vi "Gaussian-FIT.vi"() -> ()   [LabVIEW 2014]
uses:
  <vilib>/Utility/file.llb/Read From Spreadsheet File (DBL).vi
  <vilib>/Utility/file.llb/Write To Spreadsheet File (DBL).vi
  <vilib>/Analysis/NI_AALBase.lvlib
panel:
  in  "Tab Control":T1(tab)
  out "Amplitude Gaussian FIT":cluster{dbl[], dbl[]}(graph)={[6.4e-05, 5.6e-05, 4.6e-05, 6.8e-05, 7.8e-05, 7.4e-05, 9.5e-05, 0.000102, 0.000147, 0.000188, 0.000179, 0.000194, 0.000233, 0.00028, 0.000335, 0.000368, 0.000395, 0.000446, 0.000468, 0.000498, 0.000562, 0.000618, 0.000645, 0.000701, 0.000794, 0.000861, 0.000909, 0.000954, 0.001065, 0.001094, 0.001148, 0.001209, 0.0013, 0.001352, 0.001399, 0.001466, 0.001535, 0.001652, 0.001691, 0.001795, 0.001868, 0.00196, 0.00202, 0.00211, 0.00216, 0.002174, 0.002327, 0.002362, 0.002461, 0.002579, 0.002617, 0.002789, 0.002914, 0.002903, 0.003058, 0.003139, 0.003095, 0.003248, 0.003331, 0.003408, 0.003368, 0.003563, 0.003651, 0.003758, 0.003758, 0.003954, 0.003961, 0.004072, 0.004061, 0.004096, 0.004277, 0.004275, 0.004396, 0.004423, 0.004449, 0.004604, 0.004582, 0.004732, 0.004694, 0.004793, 0.004779, 0.004842, 0.004904, 0.004958, 0.004899, 0.004964, 0.005117, 0.005151, 0.005106, 0.005159, 0.005259, 0.00524, 0.005241, 0.005238, 0.005336, 0.005361, 0.005331, 0.005344, 0.005383, 0.005275, 0.00538, 0.005499, 0.005403, 0.005524, 0.00542], [82.13729352165659, 64.7849924275446, 64.78498654301572, 53.26762424681512, 53.26848684767046, 75.33492935987732, 98.57236716401128, 95.0782689280903, 106.98838926342651, 106.98830571153056, 115.68100244184599, 146.72665216048009, 163.13830277043354, 291.19836865057766, 291.1983657333123, 210.1652309953322, 210.1652442219881, 331.0652563735002, 386.4065018531679, 401.7529834685663, 430.5029627977273, 430.50296602090975, 471.5410739421762, 503.71464143125144, 517.9881482668702, 523.924898034199, 569.4214984543443, 569.4214612337393, 631.5620103806252, 655.7737694758601, 655.4855289569315, 655.4855299040236, 732.9802005633946, 766.2747596963685, 766.2747953082397, 778.1006128617066, 847.3463703094712, 878.1237605806596, 880.4301016814038, 916.1011404952861, 963.7757722908383, 990.7197405612773, 1030.0640889501683, 1030.0640536247415, 1058.8701478567225, 1058.8702047512666, 1111.6711179926594, 1111.6711847188385, 1153.6676174579575, 1235.7737499701648, 1235.773723593764, 1294.696999033421, 1332.8062134493603, 1332.8061973980577, 1409.6029130208294, 1520.9638380251768, 1502.7931626027435, 2078.3321696288353, 2130.9631611771083, 3080.5296903165968, 2867.478006984899, 3715.361825956468, 4097.6900064907, 4097.690187942468, 5707.884613662024, 8114.949905194222, 6791.547031549109, 6791.547266896523, 7366.489185680224, 10189.609439962016, 8850.977250606367, 10323.579049145412, 10393.92726685109, 13107.806221276795, 13628.609865877474, 12680.943384489134, 13203.655141195128, 16669.633175445753, 16669.633531086878, 17380.543280107122, 19592.54328706896, 17704.220065612448, 17704.21946476618, 21213.542684772063, 19802.16276737311, 24730.65246284223, 23209.70936397237, 29513.61861830476, 29513.61863160348, 22273.330376191294, 22273.32874546767, 27522.544526863705, 23565.830426930333, 26015.740961615415, 27638.42940114356, 30998.520950667462, 30998.520956690092, 34681.3207530217, 34681.32073675544, 29985.704667462593, 32493.37376081327, 34321.094245058215, 37619.55296913469, 37619.55290491994, 37256.344447207084]}
  out "Amplitude":dbl=37256.344447207084
  out "Amplitude max of Array":cluster{dbl[], dbl[]}(graph)={[6.4e-05, 5.6e-05, 4.6e-05, 6.8e-05, 7.8e-05, 7.4e-05, 9.5e-05, 0.000102, 0.000147, 0.000188, 0.000179, 0.000194, 0.000233, 0.00028, 0.000335, 0.000368, 0.000395, 0.000446, 0.000468, 0.000498, 0.000562, 0.000618, 0.000645, 0.000701, 0.000794, 0.000861, 0.000909, 0.000954, 0.001065, 0.001094, 0.001148, 0.001209, 0.0013, 0.001352, 0.001399, 0.001466, 0.001535, 0.001652, 0.001691, 0.001795, 0.001868, 0.00196, 0.00202, 0.00211, 0.00216, 0.002174, 0.002327, 0.002362, 0.002461, 0.002579, 0.002617, 0.002789, 0.002914, 0.002903, 0.003058, 0.003139, 0.003095, 0.003248, 0.003331, 0.003408, 0.003368, 0.003563, 0.003651, 0.003758, 0.003758, 0.003954, 0.003961, 0.004072, 0.004061, 0.004096, 0.004277, 0.004275, 0.004396, 0.004423, 0.004449, 0.004604, 0.004582, 0.004732, 0.004694, 0.004793, 0.004779, 0.004842, 0.004904, 0.004958, 0.004899, 0.004964, 0.005117, 0.005151, 0.005106, 0.005159, 0.005259, 0.00524, 0.005241, 0.005238, 0.005336, 0.005361, 0.005331, 0.005344, 0.005383, 0.005275, 0.00538, 0.005499, 0.005403, 0.005524, 0.00542], [161.26124644000026, 193.5661174600001, 194.12049499399996, 188.052439994, 187.1038815500002, 206.27893655000014, 214.9023718640001, 215.15528889400014, 239.98285910000016, 239.39450044600017, 243.52077844600012, 290.69092988399996, 286.0369737860001, 314.066050784, 315.1364557740003, 350.81662177400017, 350.60690978599973, 355.4613547859999, 396.0629574719999, 417.61620512000025, 449.21960901399996, 448.27930311600005, 485.6585251160001, 524.7455412300001, 534.4413229880001, 534.1995714579998, 578.1711295359999, 578.5861845659997, 653.8300735659998, 672.812892898, 667.1914465639999, 668.808947448, 760.072502448, 797.3196844379996, 798.3633899860002, 797.3925009860003, 873.8048546480001, 899.877105106, 898.7872815639998, 944.6088681139997, 981.3642943280001, 1019.0624535720001, 1060.971357664, 1060.992231784, 1088.1771207840002, 1088.534407874, 1145.5741308739998, 1145.483352786, 1187.7170187860002, 1268.7420660020002, 1268.2114752360003, 1326.707530236, 1357.539078456, 1356.7118811139999, 1559.8703811139999, 1683.961146234, 1664.65550554, 2186.310707324, 2239.269298666, 3234.030888442, 3022.4470147740003, 3763.0056222060007, 4088.9975858, 4085.75433143, 5693.3036094300005, 8105.126077335999, 6784.511360013999, 6782.972015672, 7358.951849672001, 10186.83952789, 8848.97599834, 10318.406622732, 10386.005732224, 13107.613116772, 13624.118723106, 12678.044298666, 13204.031606338, 16651.471154778003, 16650.867261876003, 17364.227872876003, 19563.959663592, 17707.432726659998, 17707.403599994, 21179.544987994, 19763.951123329996, 24694.030239784, 23186.627665368, 29478.722628468, 29479.152732235998, 22252.341288236, 22251.449526768, 27487.696026768, 23533.155386450002, 25981.78765043, 27605.285719208, 30964.39573809, 30963.588929446, 34651.51037444601, 34650.704051236, 29954.514495236, 32468.594379241997, 34291.851381780005, 37593.372641236, 37593.324096766, 37229.240762766]}
  in  "Laser Rate (Hz)":dbl=20.0
  out "Amplitude Gaussian FIT 2":cluster{dbl[], dbl[]}(graph)={[3.2e-06, 2.8e-06, 2.3e-06, 3.4e-06, 3.9e-06, 3.6999999999999997e-06, 4.75e-06, 5.1e-06, 7.35e-06, 9.4e-06, 8.949999999999999e-06, 9.7e-06, 1.165e-05, 1.3999999999999998e-05, 1.675e-05, 1.84e-05, 1.975e-05, 2.23e-05, 2.34e-05, 2.49e-05, 2.81e-05, 3.09e-05, 3.225e-05, 3.505e-05, 3.97e-05, 4.305e-05, 4.545e-05, 4.77e-05, 5.325e-05, 5.4699999999999995e-05, 5.74e-05, 6.045e-05, 6.5e-05, 6.759999999999999e-05, 6.995e-05, 7.33e-05, 7.675e-05, 8.26e-05, 8.455e-05, 8.975e-05, 9.340000000000001e-05, 9.8e-05, 0.000101, 0.00010549999999999999, 0.000108, 0.00010870000000000001, 0.00011635000000000001, 0.0001181, 0.00012305, 0.00012895000000000002, 0.00013085, 0.00013945, 0.0001457, 0.00014515, 0.0001529, 0.00015695, 0.00015475, 0.0001624, 0.00016655, 0.0001704, 0.0001684, 0.00017815000000000002, 0.00018255000000000002, 0.00018790000000000001, 0.00018790000000000001, 0.0001977, 0.00019805000000000002, 0.00020360000000000002, 0.00020305000000000003, 0.0002048, 0.00021385000000000002, 0.00021375000000000002, 0.00021979999999999998, 0.00022114999999999998, 0.00022244999999999999, 0.00023019999999999998, 0.0002291, 0.0002366, 0.0002347, 0.00023965000000000002, 0.00023895, 0.0002421, 0.0002452, 0.0002479, 0.00024494999999999996, 0.00024819999999999996, 0.00025585, 0.00025755, 0.0002553, 0.00025795, 0.00026294999999999997, 0.00026199999999999997, 0.00026205, 0.00026189999999999997, 0.0002668, 0.00026805000000000004, 0.00026655, 0.0002672, 0.00026915, 0.00026375, 0.00026900000000000003, 0.00027495000000000004, 0.00027015, 0.0002762, 0.00027100000000000003], [82.13729352165659, 64.7849924275446, 64.78498654301572, 53.26762424681512, 53.26848684767046, 75.33492935987732, 98.57236716401128, 95.0782689280903, 106.98838926342651, 106.98830571153056, 115.68100244184599, 146.72665216048009, 163.13830277043354, 291.19836865057766, 291.1983657333123, 210.1652309953322, 210.1652442219881, 331.0652563735002, 386.4065018531679, 401.7529834685663, 430.5029627977273, 430.50296602090975, 471.5410739421762, 503.71464143125144, 517.9881482668702, 523.924898034199, 569.4214984543443, 569.4214612337393, 631.5620103806252, 655.7737694758601, 655.4855289569315, 655.4855299040236, 732.9802005633946, 766.2747596963685, 766.2747953082397, 778.1006128617066, 847.3463703094712, 878.1237605806596, 880.4301016814038, 916.1011404952861, 963.7757722908383, 990.7197405612773, 1030.0640889501683, 1030.0640536247415, 1058.8701478567225, 1058.8702047512666, 1111.6711179926594, 1111.6711847188385, 1153.6676174579575, 1235.7737499701648, 1235.773723593764, 1294.696999033421, 1332.8062134493603, 1332.8061973980577, 1409.6029130208294, 1520.9638380251768, 1502.7931626027435, 2078.3321696288353, 2130.9631611771083, 3080.5296903165968, 2867.478006984899, 3715.361825956468, 4097.6900064907, 4097.690187942468, 5707.884613662024, 8114.949905194222, 6791.547031549109, 6791.547266896523, 7366.489185680224, 10189.609439962016, 8850.977250606367, 10323.579049145412, 10393.92726685109, 13107.806221276795, 13628.609865877474, 12680.943384489134, 13203.655141195128, 16669.633175445753, 16669.633531086878, 17380.543280107122, 19592.54328706896, 17704.220065612448, 17704.21946476618, 21213.542684772063, 19802.16276737311, 24730.65246284223, 23209.70936397237, 29513.61861830476, 29513.61863160348, 22273.330376191294, 22273.32874546767, 27522.544526863705, 23565.830426930333, 26015.740961615415, 27638.42940114356, 30998.520950667462, 30998.520956690092, 34681.3207530217, 34681.32073675544, 29985.704667462593, 32493.37376081327, 34321.094245058215, 37619.55296913469, 37619.55290491994, 37256.344447207084]}
  out "Amplitude max of Array 2":cluster{dbl[], dbl[]}(graph)={[3.2e-06, 2.8e-06, 2.3e-06, 3.4e-06, 3.9e-06, 3.6999999999999997e-06, 4.75e-06, 5.1e-06, 7.35e-06, 9.4e-06, 8.949999999999999e-06, 9.7e-06, 1.165e-05, 1.3999999999999998e-05, 1.675e-05, 1.84e-05, 1.975e-05, 2.23e-05, 2.34e-05, 2.49e-05, 2.81e-05, 3.09e-05, 3.225e-05, 3.505e-05, 3.97e-05, 4.305e-05, 4.545e-05, 4.77e-05, 5.325e-05, 5.4699999999999995e-05, 5.74e-05, 6.045e-05, 6.5e-05, 6.759999999999999e-05, 6.995e-05, 7.33e-05, 7.675e-05, 8.26e-05, 8.455e-05, 8.975e-05, 9.340000000000001e-05, 9.8e-05, 0.000101, 0.00010549999999999999, 0.000108, 0.00010870000000000001, 0.00011635000000000001, 0.0001181, 0.00012305, 0.00012895000000000002, 0.00013085, 0.00013945, 0.0001457, 0.00014515, 0.0001529, 0.00015695, 0.00015475, 0.0001624, 0.00016655, 0.0001704, 0.0001684, 0.00017815000000000002, 0.00018255000000000002, 0.00018790000000000001, 0.00018790000000000001, 0.0001977, 0.00019805000000000002, 0.00020360000000000002, 0.00020305000000000003, 0.0002048, 0.00021385000000000002, 0.00021375000000000002, 0.00021979999999999998, 0.00022114999999999998, 0.00022244999999999999, 0.00023019999999999998, 0.0002291, 0.0002366, 0.0002347, 0.00023965000000000002, 0.00023895, 0.0002421, 0.0002452, 0.0002479, 0.00024494999999999996, 0.00024819999999999996, 0.00025585, 0.00025755, 0.0002553, 0.00025795, 0.00026294999999999997, 0.00026199999999999997, 0.00026205, 0.00026189999999999997, 0.0002668, 0.00026805000000000004, 0.00026655, 0.0002672, 0.00026915, 0.00026375, 0.00026900000000000003, 0.00027495000000000004, 0.00027015, 0.0002762, 0.00027100000000000003], [161.26124644000026, 193.5661174600001, 194.12049499399996, 188.052439994, 187.1038815500002, 206.27893655000014, 214.9023718640001, 215.15528889400014, 239.98285910000016, 239.39450044600017, 243.52077844600012, 290.69092988399996, 286.0369737860001, 314.066050784, 315.1364557740003, 350.81662177400017, 350.60690978599973, 355.4613547859999, 396.0629574719999, 417.61620512000025, 449.21960901399996, 448.27930311600005, 485.6585251160001, 524.7455412300001, 534.4413229880001, 534.1995714579998, 578.1711295359999, 578.5861845659997, 653.8300735659998, 672.812892898, 667.1914465639999, 668.808947448, 760.072502448, 797.3196844379996, 798.3633899860002, 797.3925009860003, 873.8048546480001, 899.877105106, 898.7872815639998, 944.6088681139997, 981.3642943280001, 1019.0624535720001, 1060.971357664, 1060.992231784, 1088.1771207840002, 1088.534407874, 1145.5741308739998, 1145.483352786, 1187.7170187860002, 1268.7420660020002, 1268.2114752360003, 1326.707530236, 1357.539078456, 1356.7118811139999, 1559.8703811139999, 1683.961146234, 1664.65550554, 2186.310707324, 2239.269298666, 3234.030888442, 3022.4470147740003, 3763.0056222060007, 4088.9975858, 4085.75433143, 5693.3036094300005, 8105.126077335999, 6784.511360013999, 6782.972015672, 7358.951849672001, 10186.83952789, 8848.97599834, 10318.406622732, 10386.005732224, 13107.613116772, 13624.118723106, 12678.044298666, 13204.031606338, 16651.471154778003, 16650.867261876003, 17364.227872876003, 19563.959663592, 17707.432726659998, 17707.403599994, 21179.544987994, 19763.951123329996, 24694.030239784, 23186.627665368, 29478.722628468, 29479.152732235998, 22252.341288236, 22251.449526768, 27487.696026768, 23533.155386450002, 25981.78765043, 27605.285719208, 30964.39573809, 30963.588929446, 34651.51037444601, 34650.704051236, 29954.514495236, 32468.594379241997, 34291.851381780005, 37593.372641236, 37593.324096766, 37229.240762766]}
  out "FWHM":dbl=4.973605250619252
  out "FWHM Gaussian FIT":cluster{dbl[], dbl[]}(graph)={[6.4e-05, 5.6e-05, 4.6e-05, 6.8e-05, 7.8e-05, 7.4e-05, 9.5e-05, 0.000102, 0.000147, 0.000188, 0.000179, 0.000194, 0.000233, 0.00028, 0.000335, 0.000368, 0.000395, 0.000446, 0.000468, 0.000498, 0.000562, 0.000618, 0.000645, 0.000701, 0.000794, 0.000861, 0.000909, 0.000954, 0.001065, 0.001094, 0.001148, 0.001209, 0.0013, 0.001352, 0.001399, 0.001466, 0.001535, 0.001652, 0.001691, 0.001795, 0.001868, 0.00196, 0.00202, 0.00211, 0.00216, 0.002174, 0.002327, 0.002362, 0.002461, 0.002579, 0.002617, 0.002789, 0.002914, 0.002903, 0.003058, 0.003139, 0.003095, 0.003248, 0.003331, 0.003408, 0.003368, 0.003563, 0.003651, 0.003758, 0.003758, 0.003954, 0.003961, 0.004072, 0.004061, 0.004096, 0.004277, 0.004275, 0.004396, 0.004423, 0.004449, 0.004604, 0.004582, 0.004732, 0.004694, 0.004793, 0.004779, 0.004842, 0.004904, 0.004958, 0.004899, 0.004964, 0.005117, 0.005151, 0.005106, 0.005159, 0.005259, 0.00524, 0.005241, 0.005238, 0.005336, 0.005361, 0.005331, 0.005344, 0.005383, 0.005275, 0.00538, 0.005499, 0.005403, 0.005524, 0.00542], [67.95536302693041, 162.5803089370225, 162.58032957515317, 269.482419312964, 269.48179664269855, 167.2358722111715, 160.16237225535488, 163.72148899661636, 170.37981932006696, 170.37992665323483, 169.28782416124116, 258.1069317533028, 99.70047708647279, 102.43662819677006, 102.4366316352797, 116.74126032266032, 116.7412491941751, 102.21723891364765, 65.51556612566834, 63.72839368182466, 59.013303901778784, 59.0133030944433, 58.715195687528066, 59.602690620753876, 57.53899732335137, 59.390115972465566, 56.5072782511607, 56.50728664585086, 57.90911826225878, 56.35844407717218, 56.67232951394841, 56.672329988082936, 56.37975192843705, 56.87809918281667, 56.87809128736397, 56.020994112170094, 57.50267124417652, 56.511424488472024, 58.05385818136735, 57.515869684225564, 54.358503965363184, 58.99782921519105, 55.551829969255344, 55.55183837388944, 55.101134367999755, 55.10112470150844, 57.501970152131214, 57.50196120516605, 55.942006840849174, 57.41607411886361, 57.416079050328385, 55.97593686323666, 56.40821347852846, 56.40821703211186, 73.82063474238005, 73.27368092377942, 74.43002221748745, 55.46846389717684, 57.458464614735064, 29.536058489213104, 47.50984986559177, 12.77732110589484, 5.501323603887666, 5.50131929893884, 4.960968855647139, 5.81932949273212, 6.222341953884931, 6.222336417923118, 6.783066857597892, 5.988065634385573, 6.213856690360152, 6.190250714971343, 6.62018984759498, 6.0896176924161605, 6.4496902818501525, 6.481645777973317, 6.863052231513191, 6.31222302586826, 6.312214791553502, 6.192221142866709, 6.274846618712995, 6.480532450507895, 6.480272596126605, 6.348387561077848, 6.486231426014595, 6.296051173606955, 6.31319993031518, 5.829502928286605, 5.829502923304878, 6.253664677361324, 6.25370164540388, 6.02943489628672, 5.739455295199784, 5.834519385904765, 5.7123166397365575, 5.660175294027242, 5.660175291154464, 4.971788589692675, 4.971788595551812, 5.3312513334944285, 5.446191555161487, 5.203410464746684, 4.979688255520659, 4.979688276933952, 4.973605250619252]}
  out "FWHM Tec":cluster{dbl[], dbl[]}(graph)={[6.4e-05, 5.6e-05, 4.6e-05, 6.8e-05, 7.8e-05, 7.4e-05, 9.5e-05, 0.000102, 0.000147, 0.000188, 0.000179, 0.000194, 0.000233, 0.00028, 0.000335, 0.000368, 0.000395, 0.000446, 0.000468, 0.000498, 0.000562, 0.000618, 0.000645, 0.000701, 0.000794, 0.000861, 0.000909, 0.000954, 0.001065, 0.001094, 0.001148, 0.001209, 0.0013, 0.001352, 0.001399, 0.001466, 0.001535, 0.001652, 0.001691, 0.001795, 0.001868, 0.00196, 0.00202, 0.00211, 0.00216, 0.002174, 0.002327, 0.002362, 0.002461, 0.002579, 0.002617, 0.002789, 0.002914, 0.002903, 0.003058, 0.003139, 0.003095, 0.003248, 0.003331, 0.003408, 0.003368, 0.003563, 0.003651, 0.003758, 0.003758, 0.003954, 0.003961, 0.004072, 0.004061, 0.004096, 0.004277, 0.004275, 0.004396, 0.004423, 0.004449, 0.004604, 0.004582, 0.004732, 0.004694, 0.004793, 0.004779, 0.004842, 0.004904, 0.004958, 0.004899, 0.004964, 0.005117, 0.005151, 0.005106, 0.005159, 0.005259, 0.00524, 0.005241, 0.005238, 0.005336, 0.005361, 0.005331, 0.005344, 0.005383, 0.005275, 0.00538, 0.005499, 0.005403, 0.005524, 0.00542], [45.67945499999996, 22.588345000000004, 22.588345000000004, 43.99189899999999, 47.136563000000024, 29.512045000000057, 42.257303999999976, 57.70411100000001, 38.14522599999998, 38.14522599999998, 39.90717899999993, 46.74475400000006, 43.33263800000009, 50.22652400000004, 103.85846200000003, 42.994290999999976, 42.994290999999976, 52.29794400000003, 45.42415899999992, 44.39823100000001, 50.92581800000005, 50.92581800000005, 44.74219900000003, 54.69739800000002, 50.22652400000004, 53.340329, 50.938948000000096, 50.938948000000096, 52.99057299999993, 45.09191099999998, 48.87254699999994, 48.87254699999994, 48.87254699999994, 43.366055000000074, 46.805048000000056, 47.16082200000005, 47.86046499999998, 45.779709000000025, 47.848164999999995, 49.23496799999998, 48.54780799999992, 48.53532500000006, 46.823095999999964, 46.823095999999964, 48.54780799999992, 48.54780799999992, 49.23496799999998, 49.23496799999998, 46.13538900000003, 49.59759799999995, 49.59759799999995, 47.87889800000005, 48.578975000000014, 48.578975000000014, 45.138161999999966, 43.76056499999993, 43.76615699999991, 33.06385999999998, 36.516301999999996, 5.595047000000022, 20.228677999999945, 5.595743999999968, 4.8962759999999435, 4.8962759999999435, 4.19680900000003, 4.895667000000003, 5.24503100000004, 5.24503100000004, 5.943626999999992, 5.24503100000004, 5.24503100000004, 5.595047000000022, 5.5943509999999605, 5.24503100000004, 5.944366999999943, 5.5943509999999605, 5.943626999999992, 5.942885000000047, 5.942885000000047, 5.942885000000047, 5.942885000000047, 6.292859000000021, 6.292859000000021, 5.942885000000047, 6.292859000000021, 5.942885000000047, 5.942885000000047, 5.5929550000000745, 5.5929550000000745, 5.942885000000047, 5.942885000000047, 5.5929550000000745, 5.243068999999991, 5.5929550000000745, 5.5929550000000745, 5.243068999999991, 5.243068999999991, 4.543426000000068, 4.543426000000068, 4.893226000000027, 4.893226000000027, 4.893226000000027, 4.543426000000068, 4.543426000000068, 4.893226000000027]}
  out "FWHM Gaussian FIT 2":cluster{dbl[], dbl[]}(graph)={[3.2e-06, 2.8e-06, 2.3e-06, 3.4e-06, 3.9e-06, 3.6999999999999997e-06, 4.75e-06, 5.1e-06, 7.35e-06, 9.4e-06, 8.949999999999999e-06, 9.7e-06, 1.165e-05, 1.3999999999999998e-05, 1.675e-05, 1.84e-05, 1.975e-05, 2.23e-05, 2.34e-05, 2.49e-05, 2.81e-05, 3.09e-05, 3.225e-05, 3.505e-05, 3.97e-05, 4.305e-05, 4.545e-05, 4.77e-05, 5.325e-05, 5.4699999999999995e-05, 5.74e-05, 6.045e-05, 6.5e-05, 6.759999999999999e-05, 6.995e-05, 7.33e-05, 7.675e-05, 8.26e-05, 8.455e-05, 8.975e-05, 9.340000000000001e-05, 9.8e-05, 0.000101, 0.00010549999999999999, 0.000108, 0.00010870000000000001, 0.00011635000000000001, 0.0001181, 0.00012305, 0.00012895000000000002, 0.00013085, 0.00013945, 0.0001457, 0.00014515, 0.0001529, 0.00015695, 0.00015475, 0.0001624, 0.00016655, 0.0001704, 0.0001684, 0.00017815000000000002, 0.00018255000000000002, 0.00018790000000000001, 0.00018790000000000001, 0.0001977, 0.00019805000000000002, 0.00020360000000000002, 0.00020305000000000003, 0.0002048, 0.00021385000000000002, 0.00021375000000000002, 0.00021979999999999998, 0.00022114999999999998, 0.00022244999999999999, 0.00023019999999999998, 0.0002291, 0.0002366, 0.0002347, 0.00023965000000000002, 0.00023895, 0.0002421, 0.0002452, 0.0002479, 0.00024494999999999996, 0.00024819999999999996, 0.00025585, 0.00025755, 0.0002553, 0.00025795, 0.00026294999999999997, 0.00026199999999999997, 0.00026205, 0.00026189999999999997, 0.0002668, 0.00026805000000000004, 0.00026655, 0.0002672, 0.00026915, 0.00026375, 0.00026900000000000003, 0.00027495000000000004, 0.00027015, 0.0002762, 0.00027100000000000003], [67.95536302693041, 162.5803089370225, 162.58032957515317, 269.482419312964, 269.48179664269855, 167.2358722111715, 160.16237225535488, 163.72148899661636, 170.37981932006696, 170.37992665323483, 169.28782416124116, 258.1069317533028, 99.70047708647279, 102.43662819677006, 102.4366316352797, 116.74126032266032, 116.7412491941751, 102.21723891364765, 65.51556612566834, 63.72839368182466, 59.013303901778784, 59.0133030944433, 58.715195687528066, 59.602690620753876, 57.53899732335137, 59.390115972465566, 56.5072782511607, 56.50728664585086, 57.90911826225878, 56.35844407717218, 56.67232951394841, 56.672329988082936, 56.37975192843705, 56.87809918281667, 56.87809128736397, 56.020994112170094, 57.50267124417652, 56.511424488472024, 58.05385818136735, 57.515869684225564, 54.358503965363184, 58.99782921519105, 55.551829969255344, 55.55183837388944, 55.101134367999755, 55.10112470150844, 57.501970152131214, 57.50196120516605, 55.942006840849174, 57.41607411886361, 57.416079050328385, 55.97593686323666, 56.40821347852846, 56.40821703211186, 73.82063474238005, 73.27368092377942, 74.43002221748745, 55.46846389717684, 57.458464614735064, 29.536058489213104, 47.50984986559177, 12.77732110589484, 5.501323603887666, 5.50131929893884, 4.960968855647139, 5.81932949273212, 6.222341953884931, 6.222336417923118, 6.783066857597892, 5.988065634385573, 6.213856690360152, 6.190250714971343, 6.62018984759498, 6.0896176924161605, 6.4496902818501525, 6.481645777973317, 6.863052231513191, 6.31222302586826, 6.312214791553502, 6.192221142866709, 6.274846618712995, 6.480532450507895, 6.480272596126605, 6.348387561077848, 6.486231426014595, 6.296051173606955, 6.31319993031518, 5.829502928286605, 5.829502923304878, 6.253664677361324, 6.25370164540388, 6.02943489628672, 5.739455295199784, 5.834519385904765, 5.7123166397365575, 5.660175294027242, 5.660175291154464, 4.971788589692675, 4.971788595551812, 5.3312513334944285, 5.446191555161487, 5.203410464746684, 4.979688255520659, 4.979688276933952, 4.973605250619252]}
  out "FWHM Tec 2":cluster{dbl[], dbl[]}(graph)={[3.2e-06, 2.8e-06, 2.3e-06, 3.4e-06, 3.9e-06, 3.6999999999999997e-06, 4.75e-06, 5.1e-06, 7.35e-06, 9.4e-06, 8.949999999999999e-06, 9.7e-06, 1.165e-05, 1.3999999999999998e-05, 1.675e-05, 1.84e-05, 1.975e-05, 2.23e-05, 2.34e-05, 2.49e-05, 2.81e-05, 3.09e-05, 3.225e-05, 3.505e-05, 3.97e-05, 4.305e-05, 4.545e-05, 4.77e-05, 5.325e-05, 5.4699999999999995e-05, 5.74e-05, 6.045e-05, 6.5e-05, 6.759999999999999e-05, 6.995e-05, 7.33e-05, 7.675e-05, 8.26e-05, 8.455e-05, 8.975e-05, 9.340000000000001e-05, 9.8e-05, 0.000101, 0.00010549999999999999, 0.000108, 0.00010870000000000001, 0.00011635000000000001, 0.0001181, 0.00012305, 0.00012895000000000002, 0.00013085, 0.00013945, 0.0001457, 0.00014515, 0.0001529, 0.00015695, 0.00015475, 0.0001624, 0.00016655, 0.0001704, 0.0001684, 0.00017815000000000002, 0.00018255000000000002, 0.00018790000000000001, 0.00018790000000000001, 0.0001977, 0.00019805000000000002, 0.00020360000000000002, 0.00020305000000000003, 0.0002048, 0.00021385000000000002, 0.00021375000000000002, 0.00021979999999999998, 0.00022114999999999998, 0.00022244999999999999, 0.00023019999999999998, 0.0002291, 0.0002366, 0.0002347, 0.00023965000000000002, 0.00023895, 0.0002421, 0.0002452, 0.0002479, 0.00024494999999999996, 0.00024819999999999996, 0.00025585, 0.00025755, 0.0002553, 0.00025795, 0.00026294999999999997, 0.00026199999999999997, 0.00026205, 0.00026189999999999997, 0.0002668, 0.00026805000000000004, 0.00026655, 0.0002672, 0.00026915, 0.00026375, 0.00026900000000000003, 0.00027495000000000004, 0.00027015, 0.0002762, 0.00027100000000000003], [45.67945499999996, 22.588345000000004, 22.588345000000004, 43.99189899999999, 47.136563000000024, 29.512045000000057, 42.257303999999976, 57.70411100000001, 38.14522599999998, 38.14522599999998, 39.90717899999993, 46.74475400000006, 43.33263800000009, 50.22652400000004, 103.85846200000003, 42.994290999999976, 42.994290999999976, 52.29794400000003, 45.42415899999992, 44.39823100000001, 50.92581800000005, 50.92581800000005, 44.74219900000003, 54.69739800000002, 50.22652400000004, 53.340329, 50.938948000000096, 50.938948000000096, 52.99057299999993, 45.09191099999998, 48.87254699999994, 48.87254699999994, 48.87254699999994, 43.366055000000074, 46.805048000000056, 47.16082200000005, 47.86046499999998, 45.779709000000025, 47.848164999999995, 49.23496799999998, 48.54780799999992, 48.53532500000006, 46.823095999999964, 46.823095999999964, 48.54780799999992, 48.54780799999992, 49.23496799999998, 49.23496799999998, 46.13538900000003, 49.59759799999995, 49.59759799999995, 47.87889800000005, 48.578975000000014, 48.578975000000014, 45.138161999999966, 43.76056499999993, 43.76615699999991, 33.06385999999998, 36.516301999999996, 5.595047000000022, 20.228677999999945, 5.595743999999968, 4.8962759999999435, 4.8962759999999435, 4.19680900000003, 4.895667000000003, 5.24503100000004, 5.24503100000004, 5.943626999999992, 5.24503100000004, 5.24503100000004, 5.595047000000022, 5.5943509999999605, 5.24503100000004, 5.944366999999943, 5.5943509999999605, 5.943626999999992, 5.942885000000047, 5.942885000000047, 5.942885000000047, 5.942885000000047, 6.292859000000021, 6.292859000000021, 5.942885000000047, 6.292859000000021, 5.942885000000047, 5.942885000000047, 5.5929550000000745, 5.5929550000000745, 5.942885000000047, 5.942885000000047, 5.5929550000000745, 5.243068999999991, 5.5929550000000745, 5.5929550000000745, 5.243068999999991, 5.243068999999991, 4.543426000000068, 4.543426000000068, 4.893226000000027, 4.893226000000027, 4.893226000000027, 4.543426000000068, 4.543426000000068, 4.893226000000027]}
  out "File Analysed (output)":string="Andre-Smp-101-Spectrum mar-04-2021 Time 21-10Analysed #1.and"
  in  "Laser Rate (Hz)":dbl=20.0
  out "Array Center WL":dbl[](graph)=[577.308129, 575.915679, 575.915679, 577.308129, 577.308129, 575.915679, 578.004089, 577.308129, 578.699873, 578.699873, 575.915679, 575.915679, 575.915679, 578.004089, 578.004089, 575.915679, 575.915679, 577.308129, 580.090909, 575.915679, 578.004089, 578.004089, 577.308129, 575.915679, 575.915679, 578.004089, 578.352003, 578.352003, 577.308129, 578.004089, 579.743217, 579.743217, 577.656131, 578.004089, 578.004089, 579.047698, 578.004089, 580.090909, 577.308129, 577.308129, 579.743217, 578.004089, 578.004089, 578.004089, 577.308129, 577.308129, 577.308129, 577.308129, 576.960083, 577.308129, 577.308129, 578.699873, 580.090909, 580.090909, 563.352009, 564.051477, 563.352009, 563.352009, 563.352009, 563.352009, 563.352009, 563.352009, 563.352009, 563.352009, 563.352009, 563.701765, 563.701765, 563.701765, 563.701765, 563.701765, 563.701765, 563.352009, 563.701765, 563.701765, 563.701765, 563.701765, 563.701765, 564.401146, 564.401146, 564.750771, 565.100353, 564.051477, 564.051477, 565.449891, 565.100353, 565.449891, 564.750771, 565.449891, 565.449891, 565.100353, 565.100353, 565.449891, 565.449891, 565.449891, 565.449891, 565.799385, 565.799385, 565.799385, 565.799385, 565.449891, 565.449891, 565.799385, 565.799385, 565.799385, 565.799385]
  out "Final WL":dbl=367.780209 format="%#_3g"
  out "Initial WL":dbl=178.10648 format="%#_3g"
  in  "Length (points)":i32=500
  out "Baseline mean Chart":dbl(graph)=927.5906425599998
  out "Baseline Graph":dbl[](graph)=[884.479778, 884.479778, 884.479778, 797.099778, 782.536444, 811.905833, 780.109222, 800.497889, 790.060833, 796.371611, 775.4975, 771.371222, 787.390889, 767.973111, 815.061222, 768.458556, 781.565556, 773.798444, 797.099778, 838.848, 809.235889, 832.2945, 823.5565, 812.391278, 846.615111, 829.624556, 850.741389, 860.450278, 868.702833, 858.5085, 917.49, 924.528944, 926.228, 954.141056, 907.781111, 923.072611, 926.228, 931.082444, 914.820056, 926.470722, 927.927056, 958.024611, 948.073, 921.373556, 959.966389, 942.004944, 956.325556, 956.568278, 937.393222, 929.140667, 909.722889, 923.800778, 966.762611, 942.004944, 925.014389, 905.353889, 952.199278, 951.713833, 951.713833, 914.820056, 944.432167, 935.208722, 953.170167, 921.616278, 942.733111, 908.509278, 926.228, 927.927056, 944.432167, 913.363722, 909.965611, 980.597778, 903.654833, 925.257111, 941.276778, 927.927056, 933.752389, 935.451444, 929.868833, 926.956167, 928.897944, 904.140278, 907.538389, 943.946722, 940.305889, 935.694167, 923.800778, 944.189444, 916.761833, 913.606444, 908.023833, 923.315333, 915.548222, 928.897944, 933.024222, 932.296056, 930.111556, 920.159944, 950.985667, 930.839722, 928.655222, 904.140278, 943.946722, 958.267333, 942.490389, 912.150111, 910.693778, 941.034056, 931.082444, 954.383778, 926.470722, 965.063556, 913.363722, 938.121389, 920.888111, 930.354278, 924.771667, 899.285833, 918.218167, 946.131222, 933.752389, 990.063944, 921.859, 911.421944, 901.470333, 943.218556, 938.121389, 914.577333, 943.946722, 918.946333, 933.752389, 916.519111, 923.558056, 925.257111, 923.558056, 945.403056, 948.801167, 925.014389, 936.665056, 917.975444, 916.519111, 925.499833, 940.063167, 912.878278, 955.840111, 917.975444, 914.820056, 942.490389, 950.985667, 910.9365, 947.102111, 929.868833, 923.072611, 953.655611, 976.228778, 959.238222, 926.228, 932.296056, 938.121389, 929.140667, 954.869222, 924.286222, 933.995111, 941.034056, 914.820056, 935.694167, 921.616278, 947.102111, 930.839722, 921.130833, 932.7815, 912.392833, 930.354278, 935.694167, 923.072611, 925.257111, 920.645389, 940.305889, 925.742556, 923.315333, 967.7335, 908.752, 931.810611, 931.810611, 927.684333, 930.354278, 911.421944, 921.130833, 946.373944, 942.490389, 916.761833, 925.985278, 910.693778, 939.577722, 942.733111, 921.616278, 951.713833, 947.587556, 926.470722, 934.237833, 957.781889, 937.1505, 921.859, 926.470722, 920.159944, 920.402667, 930.354278, 965.791722, 906.5675, 934.237833, 920.159944, 952.927444, 938.849556, 923.315333, 924.528944, 912.635556, 916.276389, 911.421944, 952.199278, 949.286611, 956.082833, 947.344833, 911.179222, 943.946722, 912.392833, 932.7815, 926.228, 960.694556, 930.597, 933.266944, 926.713444, 923.558056, 917.247278, 936.179611, 914.334611, 943.218556, 911.664667, 931.567889, 908.509278, 961.18, 938.606833, 926.956167, 960.209111, 923.072611, 935.936889, 924.0435, 932.053333, 932.053333, 930.839722, 933.509667, 971.374333, 927.198889, 920.888111, 937.393222, 963.607222, 936.179611, 968.704389, 967.490778, 940.791333, 927.198889, 942.490389, 934.237833, 929.868833, 933.995111, 913.363722, 934.237833, 935.451444, 963.849944, 955.354667, 936.907778, 922.344444, 910.9365, 933.995111, 922.829889, 924.771667, 936.179611, 920.645389, 957.296444, 928.169778, 939.577722, 946.616667, 940.063167, 946.616667, 923.800778, 908.994722, 962.879056, 947.102111, 963.607222, 980.112333, 928.655222, 934.480556, 937.878667, 960.451833, 920.888111, 928.897944, 944.917611, 925.499833, 934.480556, 921.616278, 909.722889, 927.198889, 938.849556, 940.305889, 950.014778, 926.956167, 937.393222, 924.286222, 930.354278, 914.820056, 1000.986444, 929.626111, 935.208722, 917.975444, 926.470722, 943.946722, 952.199278, 911.179222, 1005.112722, 921.616278, 911.421944, 938.121389, 979.869611, 914.091889, 948.801167, 972.830667, 955.354667, 942.247667, 950.2575, 929.140667, 945.645778, 951.471111, 957.781889, 906.324778, 922.587167, 896.373167, 929.868833, 931.567889, 962.393611, 945.645778, 942.247667, 935.936889, 927.441611, 920.645389, 921.130833, 933.995111, 931.325167, 931.810611, 954.869222, 949.043889, 923.072611, 928.4125, 942.975833, 946.373944, 976.956944, 948.315722, 932.7815, 912.635556, 933.509667, 937.1505, 952.684722, 937.878667, 919.6745, 942.490389, 931.567889, 931.325167, 942.975833, 958.267333, 949.043889, 912.635556, 938.364111, 925.742556, 935.208722, 925.499833, 925.742556, 924.286222, 951.228389, 915.062778, 952.199278, 929.140667, 931.325167, 968.947111, 968.704389, 926.713444, 942.975833, 915.790944, 930.354278, 941.5195, 900.984889, 931.082444, 932.053333, 934.723278, 932.053333, 927.441611, 947.587556, 912.635556, 925.985278, 945.160333, 931.325167, 933.266944, 955.840111, 958.510056, 950.742944, 958.752778, 942.247667, 926.956167, 937.635944, 942.733111, 968.947111, 933.509667, 930.354278, 949.529333, 926.956167, 954.141056, 930.111556, 929.868833, 948.315722, 941.276778, 937.393222, 933.509667, 950.500222, 953.655611, 935.451444, 937.1505, 934.723278, 948.801167, 922.829889, 934.723278, 932.296056, 917.732722, 933.266944, 958.9955, 927.927056, 945.160333, 928.169778, 927.198889, 914.334611, 929.140667, 934.966, 919.6745, 931.082444, 925.257111, 945.645778, 941.276778, 920.402667, 918.703611, 941.276778, 930.111556, 914.577333, 929.868833, 945.403056, 933.509667, 981.811389, 944.917611, 945.403056, 953.170167, 948.801167, 934.480556, 984.238611, 964.092667, 926.956167, 932.538778, 937.878667, 922.829889, 937.393222, 932.296056, 944.917611, 956.568278, 924.771667, 907.295667, 946.131222, 920.888111, 941.5195, 924.771667, 933.266944, 945.403056, 958.267333, 975.743333, 966.519889, 942.004944, 936.179611, 953.655611, 943.704, 899.285833, 949.529333, 945.8885, 916.276389, 933.266944, 936.907778, 922.101722, 906.082056, 941.276778, 970.160722, 931.567889, 924.771667, 947.102111, 927.684333, 905.111167, 915.548222, 942.733111, 923.315333]
  out "Measures Files (in)":string="Andre-Smp-101-Measures mar-04-2021 Time 21-10.msr"
  in  "Label":string="#1"
  out "after":i32=2048
  out "before":i32=2048
  in  "Reduce Array Size (2^nTimes)":i32
  out "Gaussian FIT error":dbl[](graph)=[1041.3476751485766, 1687.7317060575303, 1687.731875392259, 1703.0143121131127, 1703.0264513314512, 2072.8613402844744, 2239.5717671729367, 2408.0812734079495, 3049.791426140287, 3049.7925619638786, 3358.508484753589, 3596.503542916978, 2055.877837984534, 4068.1966192866776, 4068.1966667575975, 4082.791141049021, 4082.7904800798888, 4983.126931226544, 2689.4537546589327, 3267.9471634315987, 2925.348025459953, 2925.348074976416, 3488.801529691946, 4325.928019906464, 4306.7485802900355, 4004.920900914679, 4325.532787811747, 4325.532392837372, 5099.711402733799, 5180.458447752411, 4574.453078521958, 4574.453062173283, 5897.825315496603, 6150.811186470055, 6150.811673274415, 6022.456337857043, 7487.045959421118, 6655.546752206932, 8817.00641524078, 8844.404657426572, 7768.935466817717, 10013.87289791547, 9655.054258754415, 9655.053412127172, 10659.695288446366, 10659.696324272607, 11984.091531483116, 11984.095771192877, 12464.974418589854, 14129.092247025068, 14129.091202263879, 13257.550166049476, 13179.327374082795, 13179.325678407726, 47216.47644861345, 52687.720637750885, 53631.41243202817, 112954.07274355332, 121595.10244613072, 155417.06256877954, 201350.4946579882, 203118.0482107672, 217468.98236445474, 217469.0081006995, 237299.9321861269, 243455.13373044555, 238204.48975080493, 238204.54491990333, 251480.3640092325, 264394.5032964509, 261930.33810224972, 297448.61289159564, 285625.280223764, 318222.6031706747, 329332.8916821739, 335016.0568371498, 385115.73007340095, 349965.40836652904, 349965.9501116744, 324121.2496453652, 316855.03193400946, 394687.4990599413, 394724.83505673875, 406075.71027588483, 320723.29267358885, 417096.04492727964, 363621.55370387726, 431523.19252474123, 431523.19215645496, 336790.44274798915, 336793.08886737213, 444572.97123484436, 360487.20184540603, 435187.0980138404, 421851.66026743915, 550319.1549059852, 550319.1550036853, 480626.3417653064, 480626.34298770357, 364032.45386185945, 391054.0373860594, 571228.8841634775, 501869.5951568715, 501869.60078787873, 556408.5388728667]
  out "time remaining (s)":string="0:00:00"
  out "%":dbl=100.0 format="%#_2f"
  out "standard deviation":dbl=13.956796655057085 format="%0.2f"
  out "Center-points":dbl[](graph)=[611.8240493028272, 611.7228207107415, 611.722817785148, 577.9552787815068, 577.9548289053191, 608.2153799765236, 605.4686324952951, 606.0823392334356, 605.2791801569227, 605.2791783994858, 604.8093028170784, 593.3434307949286, 606.6425827057122, 585.1470499277557, 585.1470504730863, 609.8707054865332, 609.8707030162768, 584.8854017957875, 584.957619122738, 582.0734512285339, 583.3377088070001, 583.3377082798258, 582.742161341459, 582.1451323465518, 581.7989391962361, 583.200866276724, 583.2255864182669, 583.2255891215556, 583.0718511652819, 583.2433227770748, 584.2180317194144, 584.2180317869177, 583.2561404763636, 583.7258169972434, 583.725814545, 584.0528567205785, 583.7464157330867, 584.7052636625372, 583.1443034351503, 583.1829524885134, 584.2044211183825, 583.9885927594343, 583.5970777488437, 583.5970807232159, 582.8899378333565, 582.8899341598485, 583.5057657022836, 583.5057612848037, 583.2843275045127, 583.4435727059976, 583.4435751273776, 584.1326670698616, 584.5627111856563, 584.5627128775341, 580.4870221070806, 581.4202909950128, 581.0288307349414, 572.625381249065, 572.9862691108784, 573.3295002033697, 574.5809305989574, 566.2111311397274, 563.4617957513981, 563.461793949283, 563.4735635267971, 563.8500612556948, 563.8582198940885, 563.8582175612423, 563.8760820048366, 563.8772690627301, 563.8728605932579, 563.5570212362306, 563.884227771169, 563.9021557461965, 563.8770000288258, 563.9006590536364, 563.9351701840873, 564.4463164111095, 564.4463129094145, 564.7739129087385, 565.058225915191, 564.0453952912943, 564.045284177915, 565.4487258363122, 564.9672640115167, 565.4491172307424, 564.7503604862046, 565.4498513150469, 565.4498513144765, 565.0595209994405, 565.0595365604162, 565.4500895422111, 565.4502746683119, 565.4498368413605, 565.4499982448812, 565.7993214142915, 565.7993214144002, 565.7993622699731, 565.7993622713572, 565.4510729408668, 565.45182690529, 565.7993376098672, 565.7993502587826, 565.799350265784, 565.7993501532909]
  out "Spectrun File (in)":string="Andre-Smp-101-Spectrum mar-04-2021 Time 21-10.spt"
  out "Powers":dbl[](graph)=[6.4e-05, 5.6e-05, 4.6e-05, 6.8e-05, 7.8e-05, 7.4e-05, 9.5e-05, 0.000102, 0.000147, 0.000188, 0.000179, 0.000194, 0.000233, 0.00028, 0.000335, 0.000368, 0.000395, 0.000446, 0.000468, 0.000498, 0.000562, 0.000618, 0.000645, 0.000701, 0.000794, 0.000861, 0.000909, 0.000954, 0.001065, 0.001094, 0.001148, 0.001209, 0.0013, 0.001352, 0.001399, 0.001466, 0.001535, 0.001652, 0.001691, 0.001795, 0.001868, 0.00196, 0.00202, 0.00211, 0.00216, 0.002174, 0.002327, 0.002362, 0.002461, 0.002579, 0.002617, 0.002789, 0.002914, 0.002903, 0.003058, 0.003139, 0.003095, 0.003248, 0.003331, 0.003408, 0.003368, 0.003563, 0.003651, 0.003758, 0.003758, 0.003954, 0.003961, 0.004072, 0.004061, 0.004096, 0.004277, 0.004275, 0.004396, 0.004423, 0.004449, 0.004604, 0.004582, 0.004732, 0.004694, 0.004793, 0.004779, 0.004842, 0.004904, 0.004958, 0.004899, 0.004964, 0.005117, 0.005151, 0.005106, 0.005159, 0.005259, 0.00524, 0.005241, 0.005238, 0.005336, 0.005361, 0.005331, 0.005344, 0.005383, 0.005275, 0.00538, 0.005499, 0.005403, 0.005524, 0.00542]
  out "Power (W)":dbl=0.00542 format="%#_6p"
  out "peak":cluster{dbl[], dbl[]}(graph)={[6.4e-05, 5.6e-05, 4.6e-05, 6.8e-05, 7.8e-05, 7.4e-05, 9.5e-05, 0.000102, 0.000147, 0.000188, 0.000179, 0.000194, 0.000233, 0.00028, 0.000335, 0.000368, 0.000395, 0.000446, 0.000468, 0.000498, 0.000562, 0.000618, 0.000645, 0.000701, 0.000794, 0.000861, 0.000909, 0.000954, 0.001065, 0.001094, 0.001148, 0.001209, 0.0013, 0.001352, 0.001399, 0.001466, 0.001535, 0.001652, 0.001691, 0.001795, 0.001868, 0.00196, 0.00202, 0.00211, 0.00216, 0.002174, 0.002327, 0.002362, 0.002461, 0.002579, 0.002617, 0.002789, 0.002914, 0.002903, 0.003058, 0.003139, 0.003095, 0.003248, 0.003331, 0.003408, 0.003368, 0.003563, 0.003651, 0.003758, 0.003758, 0.003954, 0.003961, 0.004072, 0.004061, 0.004096, 0.004277, 0.004275, 0.004396, 0.004423, 0.004449, 0.004604, 0.004582, 0.004732, 0.004694, 0.004793, 0.004779, 0.004842, 0.004904, 0.004958, 0.004899, 0.004964, 0.005117, 0.005151, 0.005106, 0.005159, 0.005259, 0.00524, 0.005241, 0.005238, 0.005336, 0.005361, 0.005331, 0.005344, 0.005383, 0.005275, 0.00538, 0.005499, 0.005403, 0.005524, 0.00542], [611.8240493028272, 611.7228207107415, 611.722817785148, 577.9552787815068, 577.9548289053191, 608.2153799765236, 605.4686324952951, 606.0823392334356, 605.2791801569227, 605.2791783994858, 604.8093028170784, 593.3434307949286, 606.6425827057122, 585.1470499277557, 585.1470504730863, 609.8707054865332, 609.8707030162768, 584.8854017957875, 584.957619122738, 582.0734512285339, 583.3377088070001, 583.3377082798258, 582.742161341459, 582.1451323465518, 581.7989391962361, 583.200866276724, 583.2255864182669, 583.2255891215556, 583.0718511652819, 583.2433227770748, 584.2180317194144, 584.2180317869177, 583.2561404763636, 583.7258169972434, 583.725814545, 584.0528567205785, 583.7464157330867, 584.7052636625372, 583.1443034351503, 583.1829524885134, 584.2044211183825, 583.9885927594343, 583.5970777488437, 583.5970807232159, 582.8899378333565, 582.8899341598485, 583.5057657022836, 583.5057612848037, 583.2843275045127, 583.4435727059976, 583.4435751273776, 584.1326670698616, 584.5627111856563, 584.5627128775341, 580.4870221070806, 581.4202909950128, 581.0288307349414, 572.625381249065, 572.9862691108784, 573.3295002033697, 574.5809305989574, 566.2111311397274, 563.4617957513981, 563.461793949283, 563.4735635267971, 563.8500612556948, 563.8582198940885, 563.8582175612423, 563.8760820048366, 563.8772690627301, 563.8728605932579, 563.5570212362306, 563.884227771169, 563.9021557461965, 563.8770000288258, 563.9006590536364, 563.9351701840873, 564.4463164111095, 564.4463129094145, 564.7739129087385, 565.058225915191, 564.0453952912943, 564.045284177915, 565.4487258363122, 564.9672640115167, 565.4491172307424, 564.7503604862046, 565.4498513150469, 565.4498513144765, 565.0595209994405, 565.0595365604162, 565.4500895422111, 565.4502746683119, 565.4498368413605, 565.4499982448812, 565.7993214142915, 565.7993214144002, 565.7993622699731, 565.7993622713572, 565.4510729408668, 565.45182690529, 565.7993376098672, 565.7993502587826, 565.799350265784, 565.7993501532909]}
  out "Current Spec":i32=105
  in  "Interactions":u32=5
  out "Total Specs":i32=105
  in  "Final":dbl=800.0
  in  "Initial":dbl=400.0
  out "Spectrum":cluster{"X Values":dbl[], "Y Values":dbl[]}[](graph)
  out "delay (ms)":u32=621
  out "peak":dbl=565.7993501532909
  # "Baseline Correct"
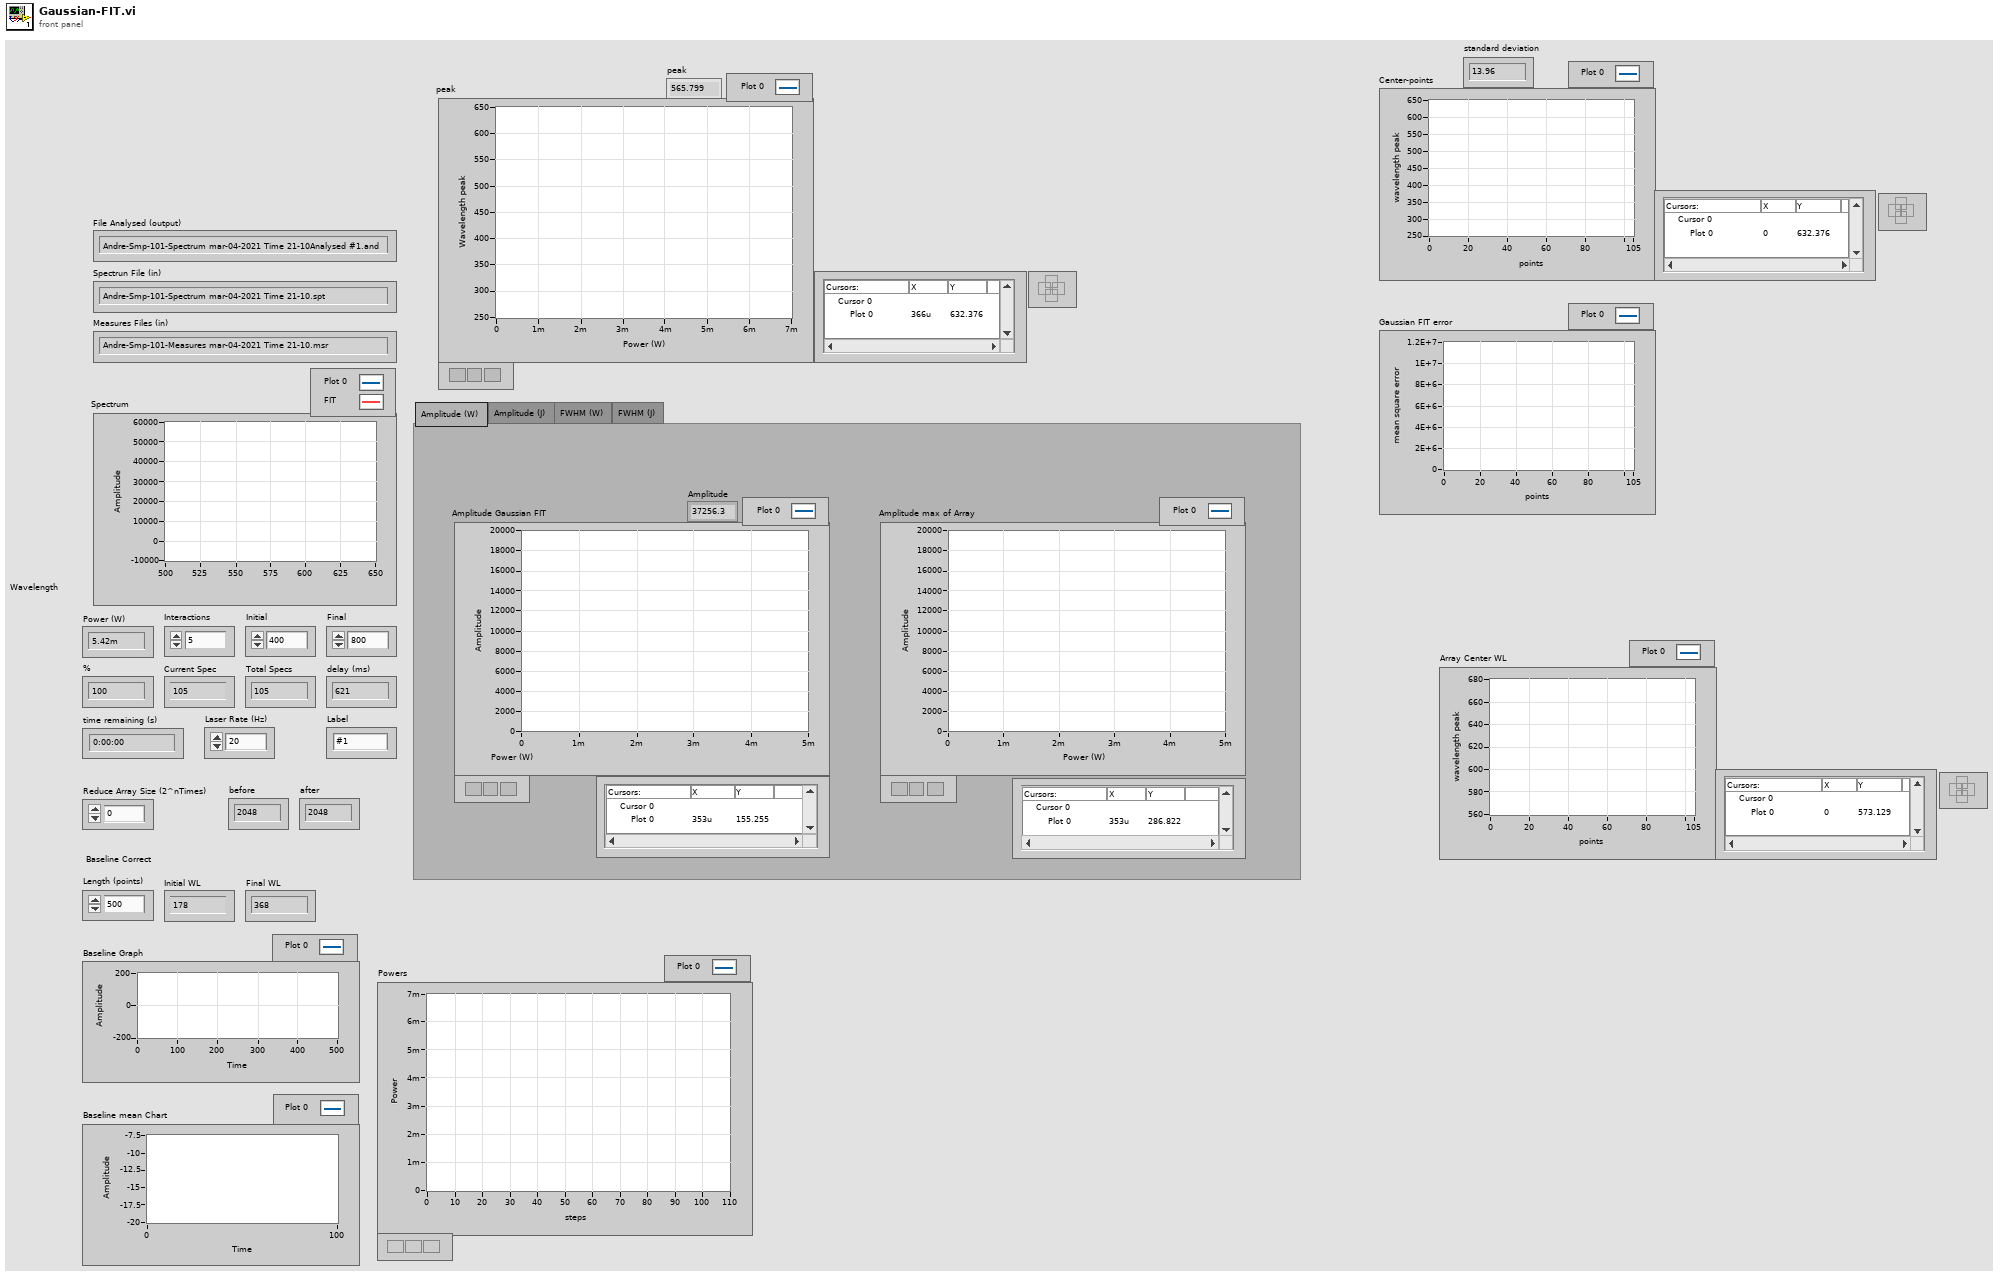
[diagram p1: front panel]
types:
  T1 = enum32{"Amplitude (W)", "Amplitude (J)", "FWHM (W)", "FWHM (J)"}
  T2 = enum16{"open", "replace", "create", "open or create", "replace or create", "replace or create with confirmation"}
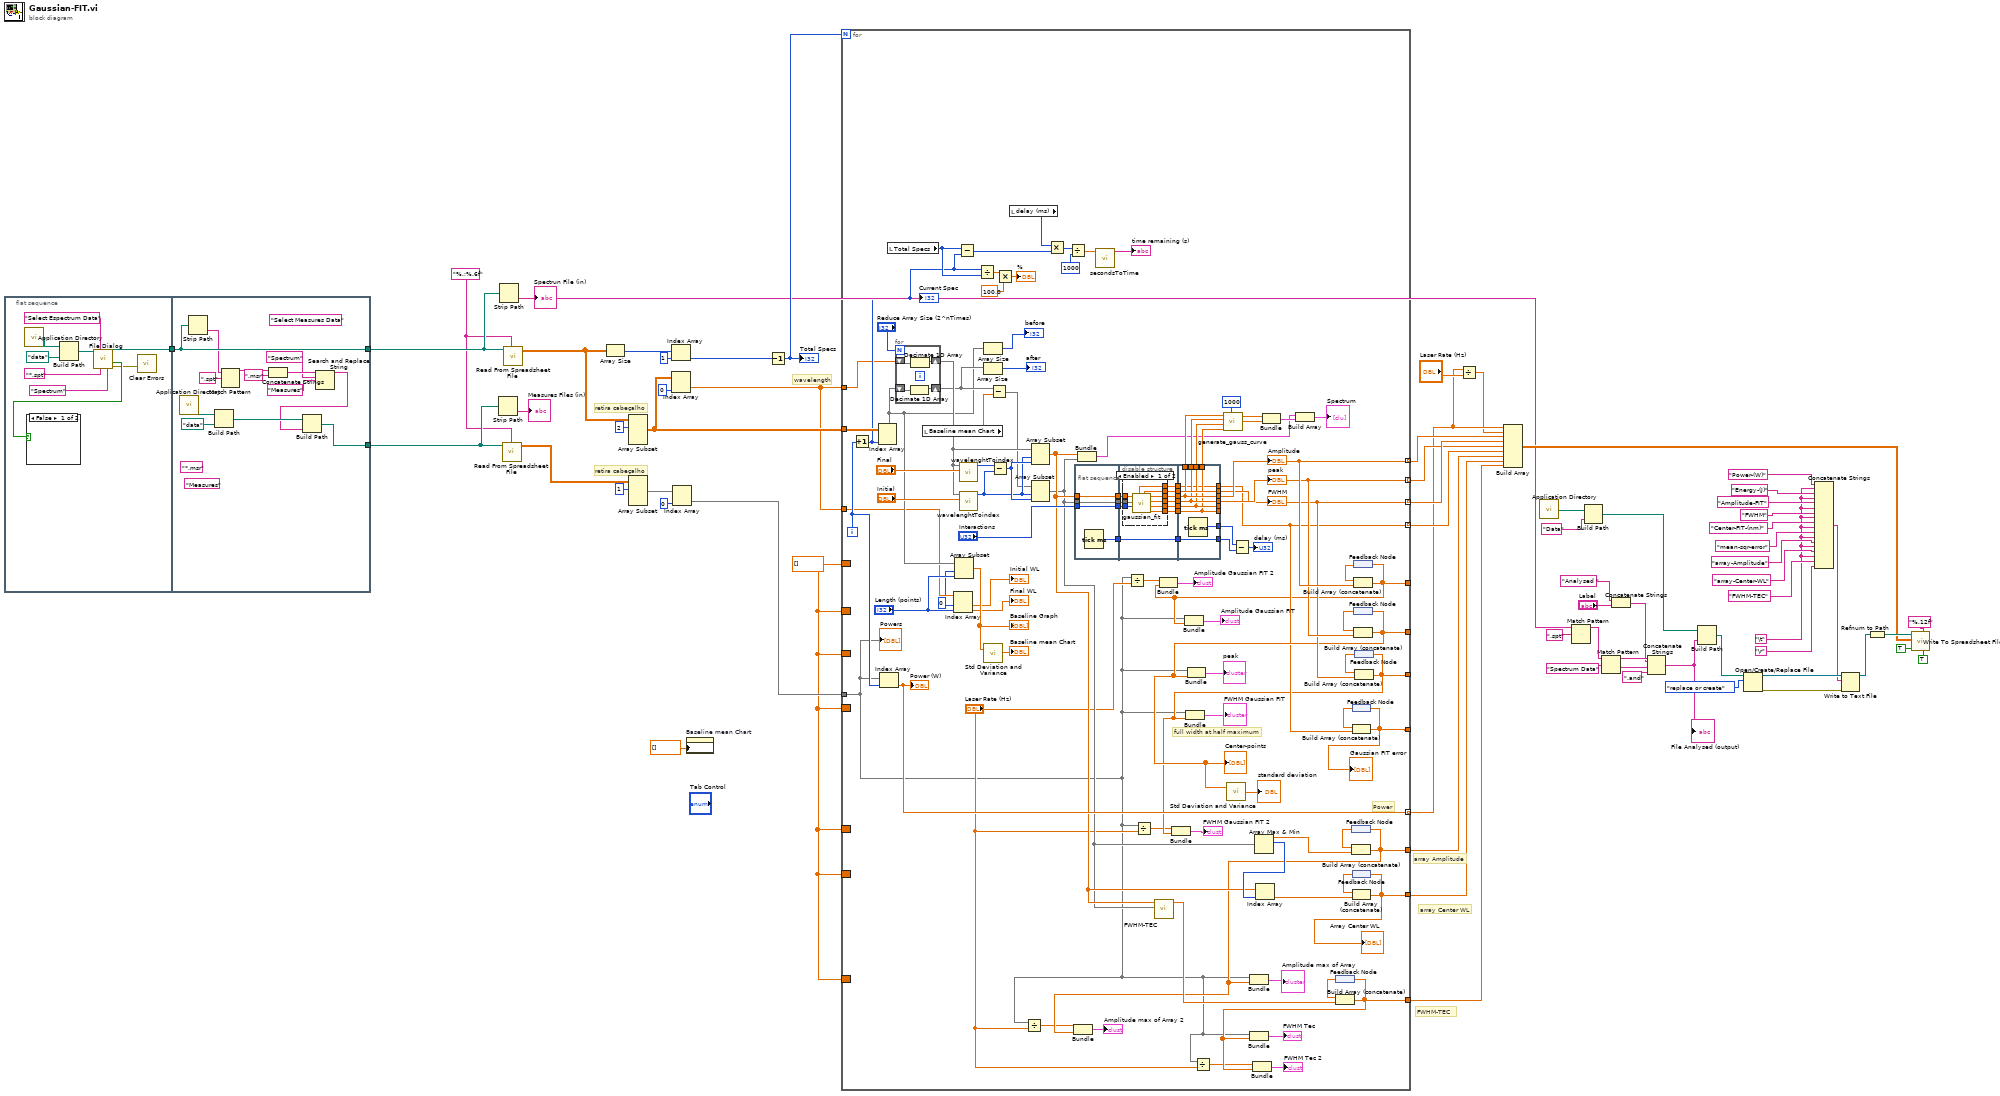
[diagram p0: block diagram]
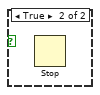
[diagram p3: hidden frame]
diagram:
  w7 = "\t"
  w15 = dbl[] []
  w1 = "%.;%.6f" ("format (%.3f)")
  # "array Amplitude"
  # "array Center WL"
  # "FWHM-TEC"
  # "wavelength"
  # "retira cabeçalho"
  # "retira cabeçalho"
  n1 = flat-sequence {
    tunnel: [w73] -> w60
    tunnel: [w87] -> w54
    tunnel: w60 -> [w87]
    tunnel: [w81] -> w19
    frame #0 {
      n2 = call <vilib>:"Application Directory.vi"() -> ("Application Directory"=w71:path)
      n3 = Build Path(base path=w71, name or relative path=path "data") -> (appended path=w70:path)
      n4 = call "File Dialog"("start path"=w70, "prompt"="Select Espectrum Data", "pattern (all files)"="*.spt", "pattern label"="Spectrum") -> ("selected path"=w73:path, "cancelled"=w69:bool, "error out"=w68:errorcluster)  [unwired: 8 in, 1 out]
      n5 = case shown="False" w69 {
        frame False {
        }
        frame True {
          n6 = Stop() -> ()  [unwired: 1 in]
        }
      }
      n7 = call <vilib>:"Clear Errors.vi"("error in (no error)"=w68) -> ()  [unwired: 5 in, 2 out]
    }
    frame #1 {
      (unwired) "Measures" ("pattern label")
      (unwired) "Select Measures Data"
      (unwired) "*.msr" ("pattern (all files)")
      n8 = call <vilib>:"Application Directory.vi"() -> ("Application Directory"=w88:path)
      n9 = Strip Path(path=w87) -> (name=w86:string)  [unwired: 1 out]
      n10 = Build Path(base path=w88, name or relative path=path "data") -> (appended path=w82:path)
      n11 = Match Pattern(string=w86, regular expression=".spt") -> (before substring=w84:string)  [unwired: 1 in, 3 out]
      n12 = Concatenate Strings(w84, ".msr" ("string")) -> (w80:string)
      n13 = Search and Replace String(input string=w80, search string="Spectrum", replace string="Measures" ("replace string (\"\")")) -> (result string=w77:string)  [unwired: 5 in, 3 out]
      n14 = Build Path(base path=w82, name or relative path=w77) -> (appended path=w81:path)
    }
  }
  n15 = Strip Path(path=w19) -> (name=→"Measures Files (in)":string)  [unwired: 1 out]
  n16 = Strip Path(path=w54) -> (name=w2:string)  [unwired: 1 out]
  "Spectrun File (in)" <- w2
  n17 = call-poly <vilib>:"Read From Spreadsheet File.vi"("format (%.3f)"=w1, "file path (dialog if empty)"=w19) -> ("all rows"=w58:dbl[][])  [unwired: 5 in, 4 out]
  n18 = call-poly <vilib>:"Read From Spreadsheet File.vi"("format (%.3f)"=w1, "file path (dialog if empty)"=w54) -> ("all rows"=w67:dbl[][])  [unwired: 5 in, 4 out]
  n19 = Array Size(array=w67) -> (size(s)=w63:i32[])
  n20 = Array Subset(array=w67, index (row)=2 ("index")) -> (w64:dbl[][])  [unwired: 3 in]
  n21 = Array Subset(array=w58, index (row)=1 ("index")) -> (w57:dbl[][])  [unwired: 3 in]
  n22 = Index Array(array=w63, index=1) -> (element=w61:i32)
  n23 = Index Array(array=w64, index (col)=0 ("disabled index (col)")) -> (element=w16:dbl[])  [unwired: 1 in]
  n24 = Index Array(array=w57, index (col)=0 ("disabled index (col)")) -> (element=w55:dbl[])  [unwired: 1 in]
  n25 = property on="Baseline mean Chart" class="WFChart (strict)"("History Data"=dbl[] []) -> ()  [unwired: 2 in, 2 out]
  n26 = Decrement(x=w61) -> (x-1=w53:i32)
  "Total Specs" <- w53
  n27 = for {
    N: w53 -> [_]
    tunnel: w16 -> [w136]
    tunnel: w64 -> [w174]
    tunnel: [w172] -> w37 mode=indexing
    tunnel: [w170] -> w30 mode=indexing
    tunnel: [w168] -> w31 mode=indexing
    border: w15 -> [_]
    tunnel: [w165] -> _
    border: w15 -> [_]
    tunnel: [w102] -> _
    border: w15 -> [_]
    tunnel: w55 -> [w91]
    tunnel: [w96] -> _
    border: w15 -> [_]
    tunnel: [w137] -> _
    tunnel: [w127] -> w4 mode=indexing
    tunnel: [w126] -> w36 mode=indexing
    tunnel: w16 -> [w119]
    border: w15 -> [_]
    tunnel: [w99] -> w10
    border: w15 -> [_]
    tunnel: [w109] -> w9
    border: w15 -> [_]
    tunnel: [w93] -> w8
    i -> [w166]
    w116 = 0 ("index")
    # "full width at half maximum"
    # "Power"
    n28 = Increment(x=w166) -> (x+1=w159:i32)
    "Current Spec" <- w159
    n29 = Index Array(array=w174, index (col)=w159) -> (element=w123:dbl[])  [unwired: 1 in]
    n30 = Index Array(array=w91, index=w166) -> (element=w127:dbl)
    "Power (W)" <- w127
    n31 = local read "Total Specs"() -> (w160:i32)
    n32 = for {
      N: "Reduce Array Size (2^nTimes)" -> [_]
      shift-right: [w191] -> w135
      shift-left: w136 -> [w193]
      shift-right: [w190] -> w134
      shift-left: w123 -> [w192]
      n33 = Decimate 1D Array(w192) -> (w190:dbl[])  [unwired: 1 out]
      n34 = Decimate 1D Array(w193) -> (w191:dbl[])  [unwired: 1 out]
    }
    n35 = local read "Baseline mean Chart"() -> (w117:dbl)
    n36 = Index Array(array=w119, index #1=w116, index #2="Length (points)") -> (element #1=→"Initial WL":dbl, element #2=→"Final WL":dbl)
    n37 = Array Subset(array=w123, index=w116, length="Length (points)") -> (w125:dbl[])
    "Baseline Graph" <- w125
    n38 = Subtract(x=w160, y=w159) -> (x-y=w156:i32)
    n39 = call "wavelenghtToindex.vi"("WL in"="Final", "WL Values"=w135) -> ("index of WL"=w176:i32)  [unwired: 9 in]
    n40 = call "wavelenghtToindex.vi"("WL in"="Initial", "WL Values"=w135) -> ("index of WL"=w175:i32)  [unwired: 9 in]
    n41 = Divide(x=w159, y=w160) -> (x/y=w163:dbl)
    n42 = Array Size(array=w134) -> (size(s)=→"after":i32)
    n43 = Array Size(array=w123) -> (size(s)=→"before":i32)
    n44 = call <vilib>:"Std Deviation and Variance.vi"("X"=w125) -> ("mean"=→"Baseline mean Chart":dbl)  [unwired: 1 in, 2 out]
    n45 = Subtract(x=w134, y=w117) -> (x-y=w118:dbl[])
    n46 = Subtract(x=w176, y=w175) -> (x-y=w177:i32)
    n47 = Multiply(x=w163, y=100.0) -> (x*y=→"%":dbl)
    n48 = local read "delay (ms)"() -> (w157:u32)
    n49 = Divide(x=w91, y="Laser Rate (Hz)") -> (x/y=w98:dbl[])
    n50 = Array Subset(array=w135, index=w175, length=w177) -> (w108:dbl[])
    n51 = Array Subset(array=w118, index=w175, length=w177) -> (w107:dbl[])
    n52 = Multiply(x=w157, y=w156) -> (x*y=w158:u32)
    n53 = Divide(x=w158, y=u32 1000 ("x")) -> (x/y=w154:dbl)
    n54 = flat-sequence {
      tunnel: w107 -> [w196]
      tunnel: w108 -> [w197]
      tunnel: [w197] -> w189
      tunnel: [w196] -> w188
      tunnel: [w195] -> w187
      tunnel: [w194] -> w186
      tunnel: "Interactions" -> [w194]
      tunnel: w189 -> [w207]
      tunnel: w188 -> [w206]
      tunnel: [w205] -> w185
      tunnel: [w204] -> w184
      tunnel: [w203] -> w183
      tunnel: w187 -> [w203]
      tunnel: w186 -> [w202]
      tunnel: [w201] -> w152
      tunnel: [w200] -> w150
      tunnel: [w199] -> w149
      tunnel: [w198] -> w139
      tunnel: [w220] -> w170
      tunnel: [w221] -> w172
      tunnel: [w224] -> w168
      tunnel: w185 -> [w221]
      tunnel: w184 -> [w220]
      tunnel: [w223] -> w182
      tunnel: [w222] -> w181
      tunnel: w183 -> [w222]
      tunnel: w152 -> [w224]
      tunnel: w150 -> [w219]
      tunnel: [w219] -> _
      tunnel: w149 -> [w218]
      tunnel: [w218] -> _
      tunnel: [w221] -> w148
      tunnel: [w220] -> w147
      tunnel: [w219] -> w146
      tunnel: [w218] -> w145
      tunnel: w139 -> [w217]
      tunnel: [w217] -> w126
      frame #0 {
        n55 = Tick Count (ms)() -> (millisecond timer value=w195:u32)
      }
      frame #1 {
        n56 = disable-structure shown="Enabled" {
          disable-tunnel: w207 -> [w216 _]
          disable-tunnel: w206 -> [w215 _]
          disable-tunnel: [w214 _] -> w205
          disable-tunnel: [w213 _] -> w204
          disable-tunnel: w202 -> [w212 _]
          disable-tunnel: [w211 _] -> w201
          disable-tunnel: [w210 _] -> w200
          disable-tunnel: [w209 _] -> w199
          disable-tunnel: [w208 _] -> w198
          frame Enabled {
            n57 = call "gaussian_fit.vi"("Max Itterations"=w212, "Y Values"=w215, "X Values"=w216) -> ("offset"=w209:dbl, "Spread (st dev)"=w210:dbl, "Center"=w213:dbl, "Amplitude"=w214:dbl, "FWHM"=w211:dbl, "mean square error"=w208:dbl)  [unwired: 1 in]
          }
          frame Disabled {
          }
        }
      }
      frame #2 {
        n58 = Tick Count (ms)() -> (millisecond timer value=w223:u32)
      }
    }
    n59 = Bundle(w108, w107) -> (w141:cluster{dbl[], dbl[]})  [unwired: 1 in]
    n60 = call "secondsToTime.vi"("Time input (s)"=w154) -> ("Time Stamp"=→"time remaining (s)":string)  [unwired: 10 in]
    n61 = Divide(x=w91, y="Laser Rate (Hz)") -> (x/y=w101:dbl[])
    n62 = Divide(x=w91, y="Laser Rate (Hz)") -> (x/y=w95:dbl[])
    n63 = call "FWHM-TEC.vi"("Y values"=w107, "WL values"=w108) -> ("FWHM"=w105:dbl)  [unwired: 9 in]
    n64 = Divide(x=w91, y="Laser Rate (Hz)") -> (x/y=w90:dbl[])
    n65 = call "generate_gauss_curve.vi"("num points"=1000, "offset"=w145, "Spread"=w146, "Center"=w147, "Amplitude"=w148) -> ("Y Values"=w143:dbl[], "X Values"=w144:dbl[])  [unwired: 3 in]
    n66 = Subtract(x=w182, y=w181) -> (x-y=→"delay (ms)":u32)
    n67 = Array Max & Min(array=w107) -> (max value=w114:dbl, max index (indices)=w112:i32)  [unwired: 2 out]
    n68 = Index Array(array=w108, index=w112) -> (element=w110:dbl)
    n69 = Bundle("X Values"=w144, "Y Values"=w143) -> (w142:cluster{"X Values":dbl[], "Y Values":dbl[]})  [unwired: 1 in]
    n70 = Build Array(w141, w142) -> (→"Spectrum":cluster{"X Values":dbl[], "Y Values":dbl[]}[])
    n71 = feedback #1() -> (w106:dbl[])
    n72 = Build Array (concatenate)(w106, w105) -> (w93:dbl[])
    n73 = Bundle(w91, w93) -> (→"FWHM Tec":cluster{dbl[], dbl[]})  [unwired: 1 in]
    n74 = Bundle(w90, w93) -> (→"FWHM Tec 2":cluster{dbl[], dbl[]})  [unwired: 1 in]
    n75 = feedback-in #1(w93) -> ()
    n76 = feedback #2() -> (w115:dbl[])
    n77 = Build Array (concatenate)(w115, w114) -> (w99:dbl[])
    n78 = Bundle(w98, w99) -> (→"Amplitude max of Array 2":cluster{dbl[], dbl[]})  [unwired: 1 in]
    n79 = Bundle(w91, w99) -> (→"Amplitude max of Array":cluster{dbl[], dbl[]})  [unwired: 1 in]
    n80 = feedback-in #2(w99) -> ()
    n81 = feedback #3() -> (w138:dbl[])
    n82 = Build Array (concatenate)(w138, w126) -> (w137:dbl[])
    "Gaussian FIT error" <- w137
    n83 = feedback-in #3(w137) -> ()
    n84 = feedback #4() -> (w111:dbl[])
    n85 = Build Array (concatenate)(w111, w110) -> (w109:dbl[])
    "Array Center WL" <- w109
    n86 = feedback-in #4(w109) -> ()
    n87 = feedback #5() -> (w173:dbl[])
    n88 = Build Array (concatenate)(w173, w172) -> (w102:dbl[])
    n89 = Bundle(w101, w102) -> (→"Amplitude Gaussian FIT 2":cluster{dbl[], dbl[]})  [unwired: 1 in]
    n90 = Bundle(w91, w102) -> (→"Amplitude Gaussian FIT":cluster{dbl[], dbl[]})  [unwired: 1 in]
    n91 = feedback-in #5(w102) -> ()
    n92 = feedback #6() -> (w171:dbl[])
    n93 = Build Array (concatenate)(w171, w170) -> (w165:dbl[])
    "Center-points" <- w165
    n94 = Bundle(w91, w165) -> (→"peak":cluster{dbl[], dbl[]})  [unwired: 1 in]
    n95 = call <vilib>:"Std Deviation and Variance.vi"("X"=w165) -> ("standard deviation"=→"standard deviation":dbl)  [unwired: 1 in, 2 out]
    n96 = feedback-in #6(w165) -> ()
    n97 = feedback #7() -> (w169:dbl[])
    n98 = Build Array (concatenate)(w169, w168) -> (w96:dbl[])
    n99 = Bundle(w95, w96) -> (→"FWHM Gaussian FIT 2":cluster{dbl[], dbl[]})  [unwired: 1 in]
    n100 = Bundle(w91, w96) -> (→"FWHM Gaussian FIT":cluster{dbl[], dbl[]})  [unwired: 1 in]
    n101 = feedback-in #7(w96) -> ()
    "FWHM" <- w168
    "Amplitude" <- w172
    "peak" <- w170
    "Powers" <- w91
  }
  n102 = Divide(x=w4, y="Laser Rate (Hz)") -> (x/y=w3:dbl[])
  n103 = Build Array(w4, w3, w37, w31, w30, w36, w10, w9, w8) -> (w34:dbl[][])
  n104 = call <vilib>:"Application Directory.vi"() -> ("Application Directory"=w41:path)
  n105 = Match Pattern(string=w2, regular expression=".spt") -> (before substring=w28:string)  [unwired: 1 in, 3 out]
  n106 = Build Path(base path=w41, name or relative path="Data" ("prompt (Create Folder)")) -> (appended path=w40:path)
  n107 = Match Pattern(string=w28, regular expression="Spectrum Data") -> (before substring=w26:string, after substring=w24:string)  [unwired: 1 in, 2 out]
  n108 = Concatenate Strings("Analysed " ("string"), "Label") -> (w22:string)
  n109 = Concatenate Strings(w26, w22, w24, ".and" ("string")) -> (w20:string)
  "File Analysed (output)" <- w20
  n110 = Build Path(base path=w40, name or relative path=w20) -> (appended path=w50:path)
  n111 = Open/Create/Replace File(file path (use dialog)=w50, operation (0:open)=T2."replace or create") -> (refnum out=w47:refnum<file>, error out=w39:errorcluster)  [unwired: 4 in, 1 out]
  n112 = Concatenate Strings("Power-(W)" ("string"), w7, "Energy-(J)" ("string"), w7, "Amplitude-FIT" ("string"), w7, "FWHM" ("string"), w7, "Center-FIT-(nm)" ("string"), w7, "mean-sqr-error" ("string"), w7, "array-Amplitude" ("string"), w7, "array-Center-WL" ("string"), w7, "FWHM-TEC" ("string"), "\r") -> (w38:string)
  n113 = Write to Text File(file (use dialog)=w47, text=w38, error in=w39) -> (refnum out=w46:refnum<file>)  [unwired: 1 in, 2 out]
  n114 = Refnum to Path(1:w46) -> (0:w52:path)
  n115 = call-poly <vilib>:"Write To Spreadsheet File.vi"("transpose? (no:F)"=TRUE, "format (%.3f)"="%.12f" ("format string"), "append to file? (new file:F)"=TRUE, "2D data"=w34, "file path (dialog if empty)"=w52) -> ()  [unwired: 3 in, 1 out]
